vi "onPublish.vi"(8 "error in (no error)":errorcluster, 10 "PUBLISH":refnum<class "PUBLISH.lvclass">, 11 "Server in":refnum<class "Server.lvclass">) -> (0 "error out":errorcluster, 3 "Server out":refnum<class "Server.lvclass">)   [LabVIEW 2013, in "MQTT Server.lvlib" / "Server.lvclass"]
uses:
  Server.lvclass
  Control Packets/PUBLISH/PUBLISH.lvclass
  MQTT_Base/MQTT_Base.lvclass
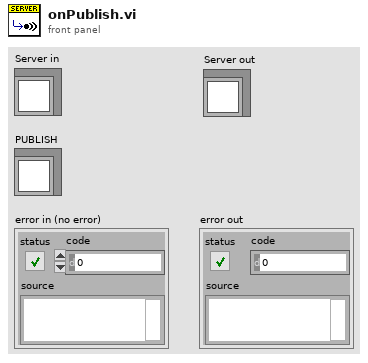
[diagram p1: front panel]
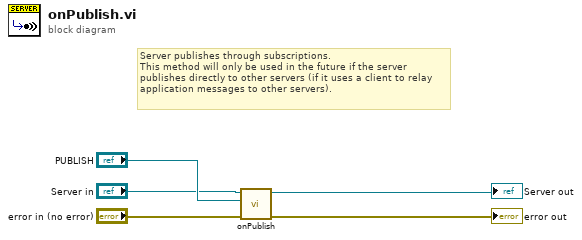
[diagram p0: block diagram]
diagram:
  # "Server publishes through subscriptions.\nThis method will only be used in the future if the server\npublishes directly to other servers (if it uses a client to relay\napplication messages to other servers)."
  n1 = call-parent "onPublish.vi"("error in (no error)"="error in (no error)", "PUBLISH"="PUBLISH", "MQTT_Base in"="Server in") -> ("error out"=→"error out":errorcluster, "MQTT_Base out"=→"Server out":refnum<class "Server.lvclass">)  [unwired: 7 in]
